vi "RT-Main.vi"() -> ()   [LabVIEW 2018]
uses:
  <vilib>/Studica/Studica Toolkit/Background/Mxp Selection.ctl
  <vilib>/robotics/Steering/Wheel/Rotation Direction.ctl
  <vilib>/robotics/Steering/Wheel/Wheel Parameters.ctl
  <vilib>/robotics/Steering/Omnidirectional Wheel/NI_Robotics_Omnidirectional Wheel.lvclass
  C:/Program Files (x86)/National Instruments/LabVIEW 2018/vi.lib/robotics/Steering/Wheel/NI_Robotics_Wheel.lvclass
  <vilib>/robotics/Steering/Omnidirectional Wheel/Create Omnidirectional Wheel.vi
  <vilib>/robotics/Steering/Steering Frame/Create User Defined Steering Frame.vi
  <vilib>/robotics/Steering/Steering Frame/Apply Steering Frame Velocity to Motors.vi
  <vilib>/robotics/Steering/Create Steering Frame/NI_Robotics_Create Steering Frame.xnode
  <vilib>/robotics/Steering/Class Type Definitions/Steering Frame.ctl
  <vilib>/robotics/Steering/Steering Frame/NI_Robotics_Steering Frame.lvclass
  <vilib>/robotics/Steering/Class Type Definitions/NI_Robotics_Steering Class Types.lvlib
  <vilib>/robotics/Steering/Wheel/NI_Robotics_Wheel.lvclass
panel:
  in  "Stop Program":bool
  in  "Robot Model":string(combo)
  out "controller data":dbl[][](array[numeric])
  out "timed out?":bool
  out "available IP addresses":string[](array[string])
  in  "Boolean":bool
  out "ccw motor velocity setpoints":dbl[](array[numeric])
  in  "Reset Encoders":bool
  out "Array of EncSpeeds":dbl[](array[numeric])
  out "Tick Count(uSec)":u32=368426469 caption="Tick Count(Ticks)"
  in  "Angular Velocity (rad/s)":dbl(slide)=-0.0 min=-1.0 max=1.0 scale=1.0..-1.0
  in  "Y Velocity (m/s)":dbl(slide)=-0.0 min=-1.0 max=1.0 scale=-1.0..1.0
  in  "X Velocity (m/s)":dbl(slide)=-0.0 min=-1.0 max=1.0 scale=-1.0..1.0
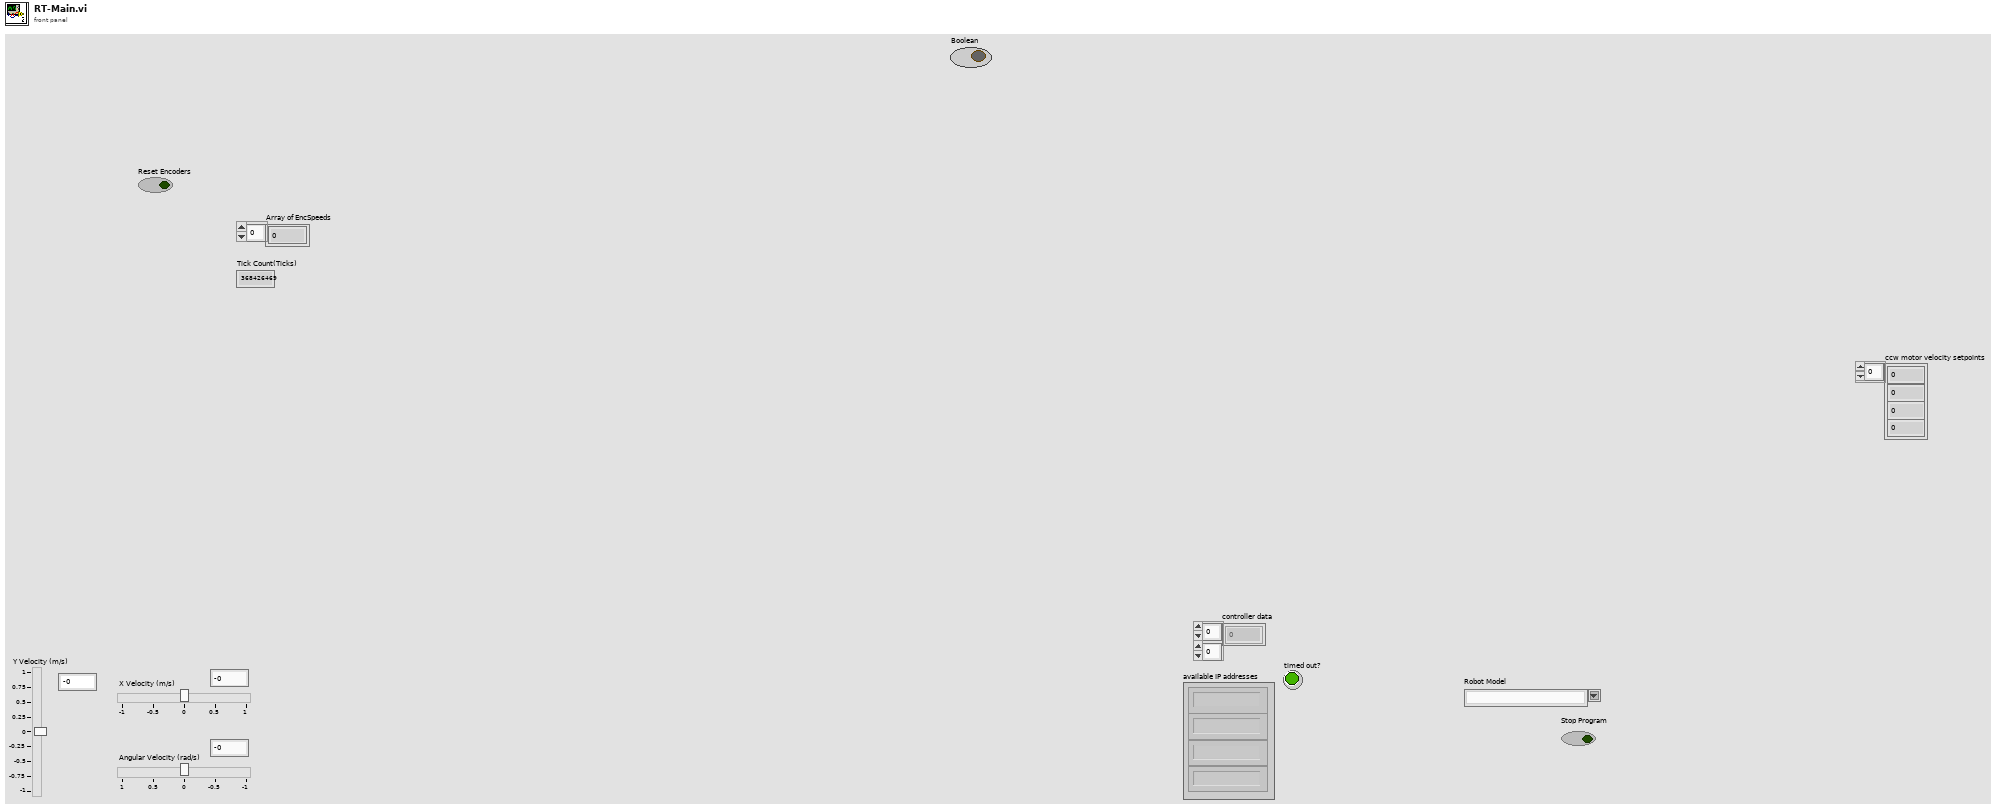
[diagram p1: front panel]
types:
  T1 = typedef "Mxp Selection.ctl" = enum16{"MXP A", "MXP B"}
  T2 = typedef "NI_Robotics_Wheel.lvclass/Wheel Parameters.ctl" = cluster{"wheel radius":dbl, "gear ratio":dbl, "forward rotation direction":T3}
  T3 = typedef "NI_Robotics_Wheel.lvclass/Rotation Direction.ctl" = u16
  T4 = typedef "NI_Robotics_Steering Class Types.lvlib/Steering Frame.ctl" = refnum<class "NI_Robotics_Steering Frame.lvclass">
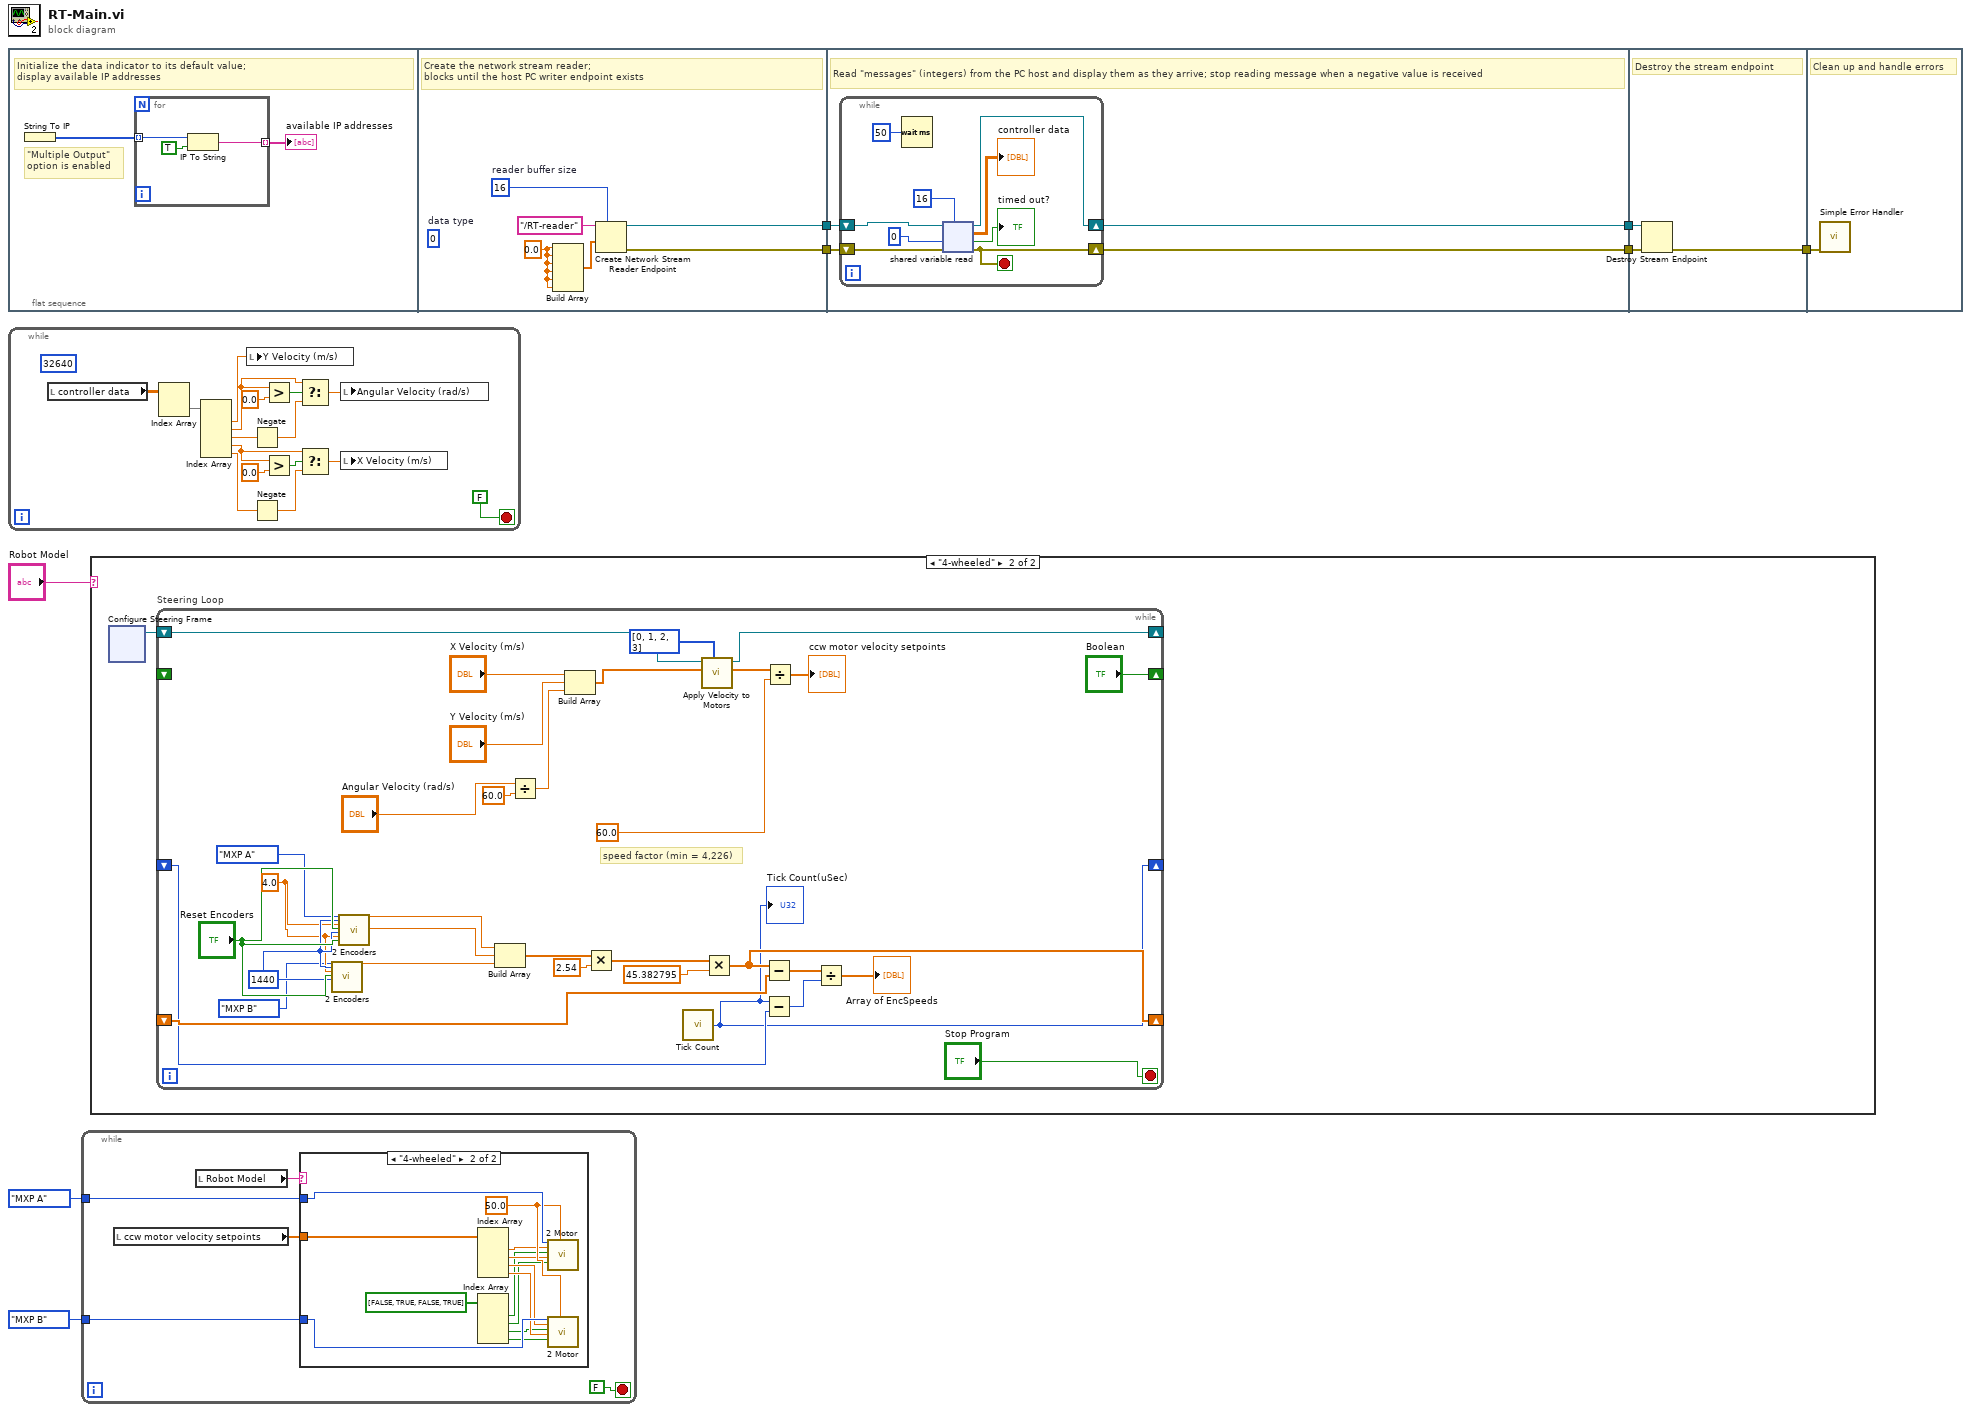
[diagram p0: block diagram]
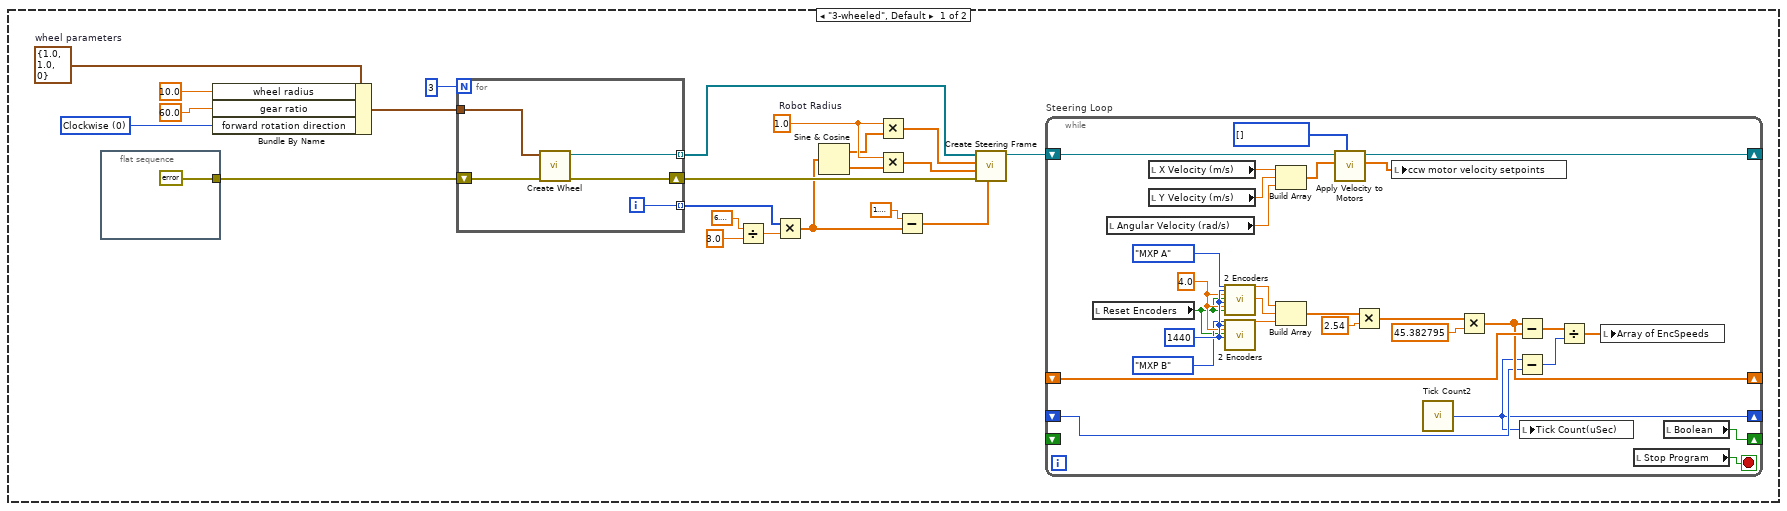
[diagram p2: hidden frame]
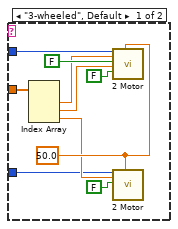
[diagram p3: hidden frame]
diagram:
  n1 = flat-sequence {
    tunnel: [w17] -> w8
    tunnel: [w16] -> w7
    tunnel: [w20] -> w6
    tunnel: [w21] -> w5
    tunnel: w8 -> [w22]
    tunnel: w7 -> [w23]
    tunnel: w6 -> [w35]
    tunnel: w5 -> [w34]
    tunnel: [w33] -> w4
    tunnel: w4 -> [w36]
    frame #0 {
      # "\"Multiple Output\"\noption is enabled"
      # "Initialize the data indicator to its default value;\ndisplay available IP addresses"
      n2 = String To IP() -> (0:w9:u32[])  [unwired: 1 in]
      n3 = for {
        tunnel: w9 -> [w12] mode=indexing
        tunnel: [w11] -> w10 mode=indexing
        n4 = IP To String(1:TRUE ("dot notation? (F)"), 2:w12) -> (0:w11:string)
      }
      "available IP addresses" <- w10
    }
    frame #1 {
      w14 = 0.0 ("element")
      (unwired) 0  # data type
      w19 = 16  # reader buffer size
      # "Create the network stream reader;\nblocks until the host PC writer endpoint exists"
      n5 = Build Array(w14, w14, w14, w14, w14, w14) -> (w15:dbl[])
      n6 = Create Network Stream Reader Endpoint(7:w19, 9:w15, 11:"/RT-reader" ("writer name")) -> (0:w17:errorcluster, 3:w16:refnum<k21>)  [unwired: 4 in]
    }
    frame #2 {
      # "Read \"messages\" (integers) from the PC host and display them as they arrive; stop reading message when a negative value is received"
      n7 = while {
        shift-right: [w30] -> w20
        shift-left: w23 -> [w32]
        shift-right: [w25] -> w21
        shift-left: w22 -> [w29]
        stop <- w25 stop-if-true
        n8 = Wait (ms)(milliseconds to wait=u32 50) -> ()  [unwired: 1 out]
        n9 = shared-variable-read(w32, w29, 0 ("timeout ms (-1)"), 16 ("# elements")) -> (w30:refnum<k21>, w25:errorcluster, →"timed out?":bool, →"controller data":dbl[][])
      }
    }
    frame #3 {
      # "Destroy the stream endpoint"
      n10 = Destroy Stream Endpoint(8:w34, 11:w35) -> (0:w33:errorcluster)
    }
    frame #4 {
      # "Clean up and handle errors"
      n11 = call <vilib>:"Simple Error Handler.vi"("error in (no error)"=w36) -> ()  [unwired: 4 in, 5 out]
    }
  }
  n12 = while {
    stop <- FALSE stop-if-true
    (unwired) 32640 ("y")
    n13 = local read "controller data"() -> (w38:dbl[][])
    n14 = Index Array(array=w38) -> (element=w45:dbl[])  [unwired: 2 in]
    n15 = Index Array(array=w45) -> (element #1=w37:dbl, element #2=w44:dbl, element #3=w43:dbl, element #4=w42:dbl, element #5=w41:dbl)  [unwired: 5 in]
    n16 = local write "Y Velocity (m/s)"(w37) -> ()
    n17 = Negate(x=w43) -> (-x=w50:dbl)
    n18 = Negate(x=w41) -> (-x=w46:dbl)
    n19 = Greater?(x=w44, y=0.0) -> (0:w52:bool)
    n20 = Greater?(x=w42, y=0.0) -> (0:w49:bool)
    n21 = Select(t=w44, s=w52, f=w50) -> (s? t:f=w40:dbl)
    n22 = Select(t=w42, s=w49, f=w46) -> (s? t:f=w47:dbl)
    n23 = local write "Angular Velocity (rad/s)"(w40) -> ()
    n24 = local write "X Velocity (m/s)"(w47) -> ()
  }
  n25 = while {
    tunnel: Mxp_Selection."MXP A" ("Mxp Side") -> [w57]
    tunnel: Mxp_Selection."MXP B" ("Mxp Side") -> [w56]
    stop <- FALSE stop-if-true
    n26 = local read "ccw motor velocity setpoints"() -> (w53:dbl[])
    n27 = local read "Robot Model"() -> (w54:string)
    n28 = case shown="\"4-wheeled\"" w54 {
      tunnel: w57 -> [w59 w80]
      tunnel: w56 -> [w58 w79]
      tunnel: w53 -> [w60 w77]
      frame "3-wheeled", Default {
        w67 = 50.0 ("Frequency [Hz]")
        n29 = Index Array(array=w60) -> (element #1=w63:dbl, element #2=w62:dbl, element #3=w61:dbl)  [unwired: 3 in]
        n30 = call <vilib>:"2 Motor.vi"("Mxp Side"=w59, "Speed M0"=w63, "Invert M0"=FALSE, "Speed M1"=w62, "Invert M1"=FALSE ("Invert M0"), "Frequency [Hz]"=w67) -> ()  [unwired: 13 in, 1 out]
        n31 = call <vilib>:"2 Motor.vi"("Mxp Side"=w58, "Speed M0"=w61, "Invert M0"=FALSE, "Frequency [Hz]"=w67) -> ()  [unwired: 15 in, 1 out]
      }
      frame "4-wheeled" {
        w78 = 50.0 ("Frequency [Hz]")
        n32 = Index Array(array=w77) -> (element #1=w76:dbl, element #2=w75:dbl, element #3=w74:dbl, element #4=w73:dbl)  [unwired: 4 in]
        n33 = Index Array(array=bool[] [FALSE, TRUE, FALSE, TRUE] ("Motor Directions")) -> (element #1=w71:bool, element #2=w70:bool, element #3=w69:bool, element #4=w68:bool)  [unwired: 4 in]
        n34 = call <vilib>:"2 Motor.vi"("Mxp Side"=w80, "Speed M0"=w76, "Invert M0"=w71, "Speed M1"=w75, "Invert M1"=w70, "Frequency [Hz]"=w78) -> ()  [unwired: 13 in, 1 out]
        n35 = call <vilib>:"2 Motor.vi"("Mxp Side"=w79, "Speed M0"=w74, "Invert M0"=w69, "Speed M1"=w73, "Invert M1"=w68, "Frequency [Hz]"=w78) -> ()  [unwired: 13 in, 1 out]
      }
    }
  }
  n36 = case shown="\"4-wheeled\"" "Robot Model" {
    frame "3-wheeled", Default {
      w102 = T2 {"wheel radius"=1.0, "gear ratio"=1.0, "forward rotation direction"=0}  # wheel parameters
      w87 = T3 0 items=["Clockwise", "Counterclockwise"] ("forward rotation direction")
      w92 = 1.0  # Robot Radius
      n37 = flat-sequence {
        tunnel: [errorcluster {"status"=FALSE, "code"=0, "source"=""} ("error out")] -> w98
        frame #0 {
        }
      }
      n38 = Bundle By Name(cluster=w102, "wheel radius"=10.0, "gear ratio"=60.0, "forward rotation direction"=w87) -> (w99:T2)
      n39 = for {
        N: 3 -> [_]
        shift-right: [w107] -> w85
        shift-left: w98 -> [w108]
        tunnel: [w106] -> w97 mode=indexing
        tunnel: w99 -> [w105]
        tunnel: [w104] -> w93 mode=indexing
        i -> [w104]
        n40 = call-poly <vilib>:"Create Wheel.vi"("error in (no error)"=w108, "wheel parameters"=w105) -> ("error out"=w107:errorcluster, "omni wheel out"=w106:refnum<class "NI_Robotics_Omnidirectional Wheel.lvclass">)  [unwired: 8 in]
      }
      n41 = Divide(x=6.283185307179586, y=3.0) -> (x/y=w94:dbl)
      n42 = Multiply(x=w93, y=w94) -> (x*y=w84:dbl[])
      n43 = Sine & Cosine(0:w84) -> (1:w83:dbl[], 2:w82:dbl[])
      n44 = Multiply(x=w92, y=w83) -> (x*y=w91:dbl[])
      n45 = Multiply(x=w92, y=w82) -> (x*y=w90:dbl[])
      n46 = Subtract(x=1.5707963267948966, y=w84) -> (x-y=w88:dbl[])
      n47 = call-poly <vilib>:"Create Steering Frame.vi"("wheel frame angles (rad)"=w88, "error in (no error)"=w85, "wheel y positions"=w90, "wheel x positions"=w91, "wheels"=w97) -> ("steering frame out"=w81:refnum<class "NI_Robotics_Steering Frame.lvclass">)  [unwired: 5 in, 1 out]
      n48 = while "Steering Loop" {
        shift-right: [w109] -> _
        shift-left: _ -> [_]
        shift-right: [w136] -> _
        shift-left: w81 -> [w137]
        shift-right: [w116] -> _
        shift-left: _ -> [w119]
        shift-right: [w120] -> _
        shift-left: _ -> [w121]
        stop <- w118 stop-if-true
        w124 = 4.0 ("Wheel Diameter M1 (inches)")
        w125 = u32 1440 ("Ticks Per Rev M0")
        n49 = local read "Reset Encoders"() -> (w113:bool)
        n50 = local read "Angular Velocity (rad/s)"() -> (w111:dbl)
        n51 = local read "X Velocity (m/s)"() -> (w112:dbl)
        n52 = local read "Y Velocity (m/s)"() -> (w110:dbl)
        n53 = call <vilib>:"2 Encoders.vi"("Mxp Side"=Mxp_Selection."MXP A", "Ticks Per Rev M0"=w125, "Wheel Diameter M0 (inches)"=w124, "Reset Encoder 0"=w113, "Ticks Per Rev M1"=w125, "Wheel Diameter M1 (inches)"=w124, "Reset Encoder 1"=w113) -> ("Distance M0 (inches)"=w126:dbl, "Distance M1 (inches)"=w127:dbl)  [unwired: 18 in, 1 out]
        n54 = call <vilib>:"2 Encoders.vi"("Mxp Side"=Mxp_Selection."MXP B", "Ticks Per Rev M0"=w125, "Wheel Diameter M0 (inches)"=w124, "Reset Encoder 0"=w113, "Ticks Per Rev M1"=w125) -> ("Distance M0 (inches)"=w128:dbl)  [unwired: 20 in, 2 out]
        n55 = Build Array(w112, w110, w111) -> (w135:dbl[])
        n56 = Build Array(w126, w127, w128) -> (w130:dbl[])
        n57 = call-poly <vilib>:"Apply Velocity to Motors.vi"("wheel indexes"=i32[] [], "steering frame velocity"=w135, "steering frame in"=w137) -> ("ccw motor velocity setpoints"=w115:dbl[], "steering frame out"=w136:refnum<class "NI_Robotics_Steering Frame.lvclass">)  [unwired: 4 in, 3 out]
        n58 = Multiply(x=w130, y=2.54) -> (x*y=w131:dbl[])
        n59 = local write "ccw motor velocity setpoints"(w115) -> ()
        n60 = call "Tick Count2"() -> ("Tick Count(uSec)"=w116:u32)
        n61 = Multiply(x=w131, y=45.382795) -> (x*y=w120:dbl[])
        n62 = Subtract(x=w120, y=w121) -> (x-y=w133:dbl[])
        n63 = Subtract(x=w116, y=w119) -> (x-y=w134:u32)
        n64 = local write "Tick Count(uSec)"(w116) -> ()
        n65 = Divide(x=w133, y=w134) -> (x/y=w117:dbl[])
        n66 = local write "Array of EncSpeeds"(w117) -> ()
        n67 = local read "Stop Program"() -> (w118:bool)
        n68 = local read "Boolean"() -> (w109:bool)
      }
    }
    frame "4-wheeled" {
      n69 = xnode ("Configure Steering Frame")() -> ("steering frame out"=w138:T4)  [unwired: 1 in, 1 out]
      n70 = while "Steering Loop" {
        shift-right: ["Boolean"] -> _
        shift-left: _ -> [_]
        shift-right: [w192] -> _
        shift-left: w138 -> [w193]
        shift-right: [w172] -> _
        shift-left: _ -> [w173]
        shift-right: [w174] -> _
        shift-left: _ -> [w175]
        stop <- "Stop Program" stop-if-true
        w179 = 4.0 ("Wheel Diameter M1 (inches)")
        w180 = u32 1440 ("Ticks Per Rev M0")
        # "speed factor (min = 4,226)"
        n71 = call <vilib>:"2 Encoders.vi"("Mxp Side"=Mxp_Selection."MXP B", "Ticks Per Rev M0"=w180, "Wheel Diameter M0 (inches)"=w179, "Reset Encoder 0"="Reset Encoders", "Ticks Per Rev M1"=w180) -> ("Distance M0 (inches)"=w184:dbl)  [unwired: 20 in, 2 out]
        n72 = call <vilib>:"2 Encoders.vi"("Mxp Side"=Mxp_Selection."MXP A", "Ticks Per Rev M0"=w180, "Wheel Diameter M0 (inches)"=w179, "Reset Encoder 0"="Reset Encoders", "Ticks Per Rev M1"=w180, "Wheel Diameter M1 (inches)"=w179, "Reset Encoder 1"="Reset Encoders") -> ("Distance M0 (inches)"=w182:dbl, "Distance M1 (inches)"=w183:dbl)  [unwired: 18 in, 1 out]
        n73 = Build Array(w182, w183, w184) -> (w186:dbl[])
        n74 = Divide(x="Angular Velocity (rad/s)", y=60.0) -> (x/y=w162:dbl)
        n75 = Build Array("X Velocity (m/s)", "Y Velocity (m/s)", w162) -> (w191:dbl[])
        n76 = Multiply(x=w186, y=2.54) -> (x*y=w187:dbl[])
        n77 = call "Tick Count"() -> ("Tick Count(uSec)"=w172:u32)
        "Tick Count(uSec)" <- w172
        n78 = call-poly <vilib>:"Apply Velocity to Motors.vi"("wheel indexes"=i32[] [0, 1, 2, 3], "steering frame velocity"=w191, "steering frame in"=w193) -> ("ccw motor velocity setpoints"=w167:dbl[], "steering frame out"=w192:T4)  [unwired: 4 in, 3 out]
        n79 = Multiply(x=w187, y=45.382795) -> (x*y=w174:dbl[])
        n80 = Subtract(x=w174, y=w175) -> (x-y=w189:dbl[])
        n81 = Subtract(x=w172, y=w173) -> (x-y=w190:u32)
        n82 = Divide(x=w167, y=60.0 ("Wheel Diameter M1 (inches)")) -> (x/y=→"ccw motor velocity setpoints":dbl[])
        n83 = Divide(x=w189, y=w190) -> (x/y=→"Array of EncSpeeds":dbl[])
      }
    }
  }
